vi "NI6000_DO_SA.vi"() -> ()   [LabVIEW 2012]
uses:
  <vilib>/DAQmx/write.llb/DAQmx Write (Digital 1D Bool NChan 1Samp 1Line).vi
  <vilib>/DAQmx/miscellaneous.llb/DAQmx Fill In Error Info.vi
  H2O_DIAL/LabVIEW-2012/Bristol WM V2_31b/CLDevIFace.dll
panel:
  in  "Bristol In":i32=5
  out "Lambda":dbl format="%.6g"
  out "Bristol Out":i32=1
  in  "STOP":bool
  out "error out":errorcluster
  in  "Line 3":bool
  in  "Line 2":bool
  in  "Line 1":bool
  in  "Line 0":bool=TRUE
  # "NI6000 Digital Out"
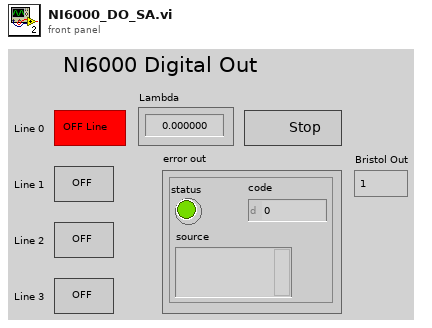
[diagram p1: front panel]
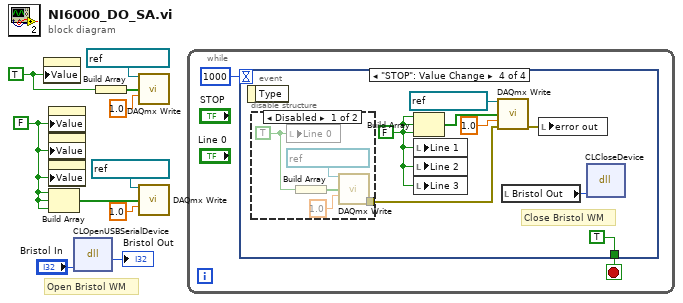
[diagram p0: block diagram]
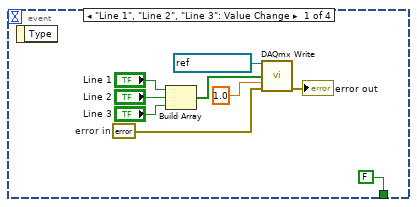
[diagram p2: hidden frame]
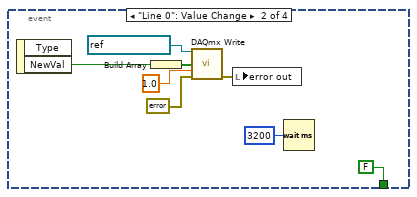
[diagram p3: hidden frame]
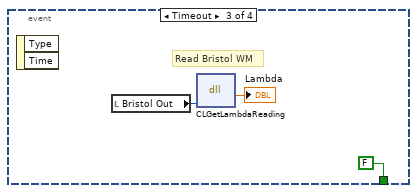
[diagram p4: hidden frame]
diagram:
  w6 = FALSE ("Line 0")
  w2 = TRUE ("Line 0")
  # "Open Bristol WM"
  n1 = property on="Line 0" class="Bool (strict)"("Value"=w2) -> ()  [unwired: 2 in, 2 out]
  n2 = property on="Line 1" class="Bool (strict)"("Value"=w6) -> ()  [unwired: 2 in, 2 out]
  n3 = property on="Line 2" class="Bool (strict)"("Value"=w6) -> ()  [unwired: 2 in, 2 out]
  n4 = property on="Line 3" class="Bool (strict)"("Value"=w6) -> ()  [unwired: 2 in, 2 out]
  n5 = Build Array(w6, w6, w6) -> (w7:bool[])
  n6 = dll-call lib="C:/H2O_DIAL/LabVIEW-2012/Bristol WM V2_31b/CLDevIface.dll" fn="CLOpenUSBSerialDevice"("commPort"="Bristol In") -> ("return type"=→"Bristol Out":i32)  [unwired: 4 in, 2 out]
  n7 = Build Array(w2) -> (w3:bool[])
  n8 = call-poly <vilib>:"DAQmx Write.vi"("task/channels in"=refnum<k21> "BristolWM", "data"=w3, "timeout"=1.0) -> ()  [unwired: 10 in, 3 out]
  n9 = call-poly <vilib>:"DAQmx Write.vi"("task/channels in"=refnum<k21> "ThreeDIO" ("ThreeDIO"), "data"=w7, "timeout"=1.0) -> ()  [unwired: 10 in, 3 out]
  n10 = while {
    stop <- w12 stop-if-true
    n11 = event shown="[3] \"STOP\": Value Change" {
      selector: _ -> [_ _ _ _]
      dyn-events: _ -> [_ _ _ _]
      timeout: 1000 -> [_ _ _ _]
      tunnel: [FALSE FALSE FALSE TRUE] -> w12
      event "Line 1", "Line 2", "Line 3": Value Change {
        w15 = errorcluster {"status"=FALSE, "code"=0, "source"=""}  # error in
        n12 = event-data() -> ()  [unwired: 1 in, 1 out]
        n13 = Build Array("Line 1", "Line 2", "Line 3") -> (w18:bool[])
        n14 = call-poly <vilib>:"DAQmx Write.vi"("task/channels in"=refnum<k21> "ThreeDIO", "data"=w18, "timeout"=1.0, "error in"=w15) -> ("error out"=→"error out":errorcluster)  [unwired: 9 in, 2 out]
      }
      event "Line 0": Value Change {
        n15 = event-data() -> ("NewVal"=w26:bool)  [unwired: 1 in, 1 out]
        n16 = Build Array(w26) -> (w25:bool[])
        n17 = call-poly <vilib>:"DAQmx Write.vi"("task/channels in"=refnum<k21> "BristolWM", "data"=w25, "timeout"=1.0, "error in"=errorcluster {"status"=FALSE, "code"=0, "source"=""}) -> ("error out"=w23:errorcluster)  [unwired: 9 in, 2 out]
        n18 = local write "error out"(w23) -> ()
        n19 = Wait (ms)(milliseconds to wait=u32 3200) -> ()  [unwired: 1 out]
      }
      event Timeout {
        # "Read Bristol WM"
        n20 = event-data() -> ()  [unwired: 1 in, 2 out]
        n21 = local read "Bristol Out"() -> (w32:i32)
        n22 = dll-call lib="C:/H2O_DIAL/LabVIEW-2012/Bristol WM V2_31b/CLDevIface.dll" fn="CLGetLambdaReading"("devHandle"=w32) -> ("return type"=→"Lambda":dbl)  [unwired: 4 in, 2 out]
      }
      event "STOP": Value Change {
        w35 = FALSE
        # "Close Bristol WM"
        n23 = event-data() -> ()  [unwired: 1 in, 1 out]
        n24 = disable-structure shown="Disabled" {
          disable-tunnel: [w41 _] -> w33
          frame Disabled {
            w42 = TRUE
            n25 = local write "Line 0"(w42) -> ()
            n26 = Build Array(w42) -> (w44:bool[])
            n27 = call-poly <vilib>:"DAQmx Write.vi"("task/channels in"=refnum<k21> "BristolWM", "data"=w44, "timeout"=1.0) -> ("error out"=w41:errorcluster)  [unwired: 10 in, 2 out]
          }
          frame Enabled {
          }
        }
        n28 = Build Array(w35, w35, w35) -> (w37:bool[])
        n29 = local write "Line 1"(w35) -> ()
        n30 = local write "Line 2"(w35) -> ()
        n31 = local write "Line 3"(w35) -> ()
        n32 = call-poly <vilib>:"DAQmx Write.vi"("task/channels in"=refnum<k21> "ThreeDIO", "data"=w37, "timeout"=1.0, "error in"=w33) -> ("error out"=w36:errorcluster)  [unwired: 9 in, 2 out]
        n33 = local read "Bristol Out"() -> (w39:i32)
        n34 = local write "error out"(w36) -> ()
        n35 = dll-call lib="C:/H2O_DIAL/LabVIEW-2012/Bristol WM V2_31b/CLDevIFace.dll" fn="CLCloseDevice"("CommPort"=w39) -> ()  [unwired: 5 in, 2 out]
      }
    }
  }
